vi "DAC Run.vi"(8 "error in":errorcluster, 11 "DAC RTD Temp in":refnum<class "DAC RTD Temp.lvclass">) -> (0 "error out":errorcluster, 3 "DAC RTD Temp out":refnum<class "DAC RTD Temp.lvclass">)   [LabVIEW 2019, in "DAC.lvlib" / "DAC RTD Temp.lvclass"]
uses:
  DAC RTD Temp.lvclass
  DAC.lvclass
  C:/Users/wg/Documents/LV_Projects/test-stand/App/DAC/DAC.lvclass
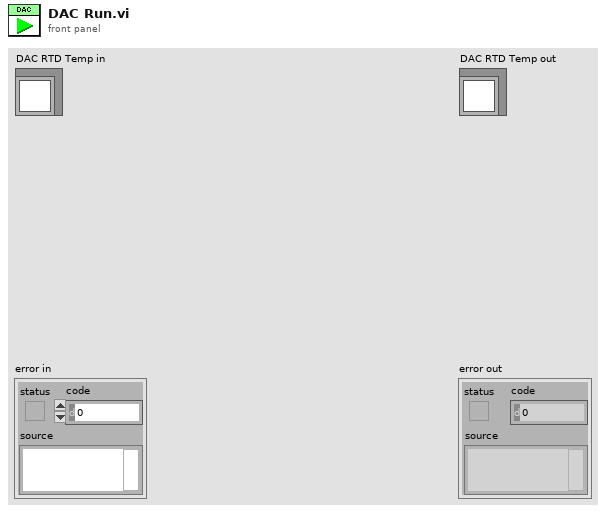
[diagram p1: front panel]
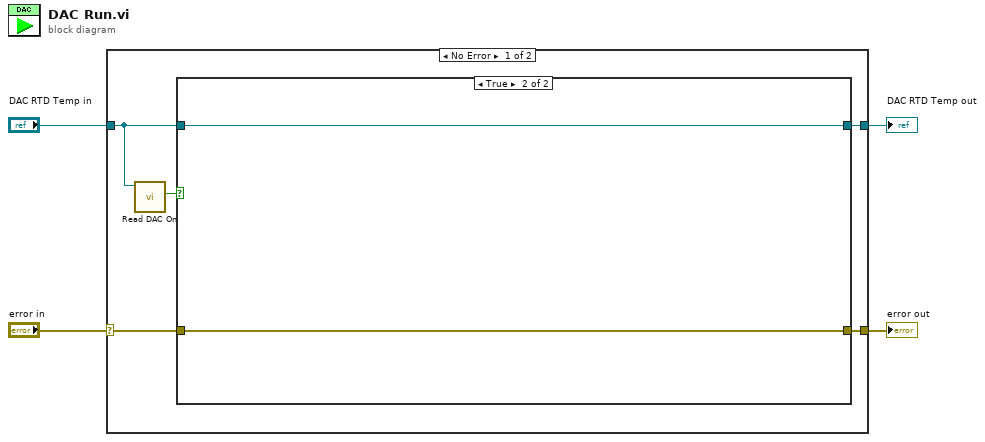
[diagram p0: block diagram]
diagram:
  n1 = case shown="No Error" "error in" {
    selector: "error in" -> [w7 w15]
    tunnel: [w6 w15] -> w2
    tunnel: [w8 w14] -> w1
    tunnel: "DAC RTD Temp in" -> [w5 w14]
    frame No Error {
      n2 = call "Read DAC On.vi"("DAC in"=w5) -> ("DAC On"=w9:bool)  [unwired: 8 in, 2 out]
      n3 = case shown="True" w9 {
        tunnel: w5 -> [w11 w13]
        tunnel: [w11 w13] -> w8
        tunnel: w7 -> [w10 w12]
        tunnel: [w10 w12] -> w6
        frame False {
        }
        frame True {
        }
      }
    }
    frame Error {
    }
  }
  "error out" <- w2
  "DAC RTD Temp out" <- w1
